vi "Lift Control (SubVI).vi"(10 "Buttons":bool[](array[boolean]), 11 "Lift PID gains":T1={"proportional gain (Kc)"=1.0, "integral time (Ti, min)"=0.01, "derivative time (Td, min)"=0.0} {"derivative time (Td, min)" format="%.3f"; "integral time (Ti, min)" format="%.3f"; "proportional gain (Kc)" format="%.3f"}) -> ()   [LabVIEW 2014]
uses:
  <vilib>/Rock Robotics/WPI/Solenoid/WPI_SolenoidValue.ctl
  <vilib>/Rock Robotics/WPI/Solenoid/WPI_SolenoidSetEnum.vi
  <vilib>/addons/control/pid/pid.llb/PID (DBL).vi
  <vilib>/addons/control/pid/NI_PID_pid.lvlib
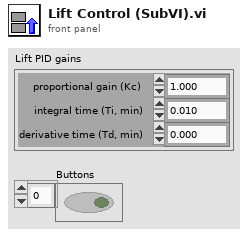
[diagram p1: front panel]
types:
  T1 = cluster{"proportional gain (Kc)":dbl, "integral time (Ti, min)":dbl, "derivative time (Td, min)":dbl}
  T2 = typedef "WPI_SolenoidValue.ctl" = enum16{"Off", "On", "Forward", "Reverse"}
  T3 = typedef "WPI_EncoderDevRef.ctl" = cluster{"DevStatus":errorcluster, "EncoderIndex":T4, "CounterIndex":T5, "DistancePerCount":dbl, "Decoding Type":T6}
  T4 = typedef "FPGA_EncoderIdx.ctl" = enum8{"Enc 0", "Enc 1", "Enc 2", "Enc 3", "Enc 4", "Enc 5", "Enc 6", "Enc 7", "Invalid"}
  T5 = typedef "FPGA_CounterCtrSystemIndex.ctl" = enum8{"Ctr 0", "Ctr 1", "Ctr 2", "Ctr 3", "Ctr 4", "Ctr 5", "Ctr 6", "Ctr 7", "Invalid"}
  T6 = typedef "WPI_EncoderType.ctl" = enum16{"1x", "2x", "4x"}
  T7 = typedef "WPI_SolenoidDevRef.ctl" = cluster{"DevStatus":errorcluster, "Pneumatics Control Module":u8, "Forward Solenoid Channel":T8, "Reverse Solenoid Channel":T8}
  T8 = typedef "WPI_SolenoidChannel.ctl" = enum8{"Solenoid 0", "Solenoid 1", "Solenoid 2", "Solenoid 3", "Solenoid 4", "Solenoid 5", "Solenoid 6", "Solenoid 7", "Invalid"}
  T9 = typedef "WPI_SwitchDevRef.ctl" = cluster{"DevStatus":errorcluster, "DIO Channel":T10, "Controller":T11, "CntIndex":T5, "Normally Closed":bool}
  T10 = typedef "FPGA_DIOChannel.ctl" = enum8{"DIO 0", "DIO 1", "DIO 2", "DIO 3", "DIO 4", "DIO 5", "DIO 6", "DIO 7", "DIO 8", "DIO 9", "DIO MXP 0", "DIO MXP 1", "DIO MXP 2", "DIO MXP 3", "DIO MXP 4", "DIO MXP 5", "DIO MXP 6", "DIO MXP 7", "DIO MXP 8", "DIO MXP 9", "DIO MXP 10", "DIO MXP 11", "DIO MXP 12", "DIO MXP 13", "DIO MXP 14", "DIO MXP 15", "Invalid"}
  T11 = typedef "FPGA_TypedefDigitalModule.ctl" = enum16{"Controller 1"}
  T12 = typedef "WPI_MotorControlDeviceRef.ctl" = cluster{"DeviceStatus":errorcluster, "Type":T13, "PWM":cluster{"Controller":T11, "PWM Channel":T14, "DeadBand":T15}, "CAN":cluster{"Device Number":u8, "Control Mode":T16, "Semaphore":T17, "Max Vout":dbl, "TalonSRX Control Mode":T18}, "Invert":bool, "TransformRef":T19, "InvTransformRef":T19}
  T13 = typedef "WPI_MotorControlType.ctl" = enum16{"PWM", "CAN", "CANTalonSRX"}
  T14 = typedef "FPGA_DIOPWMChannel.ctl" = enum8{"PWM 0", "PWM 1", "PWM 2", "PWM 3", "PWM 4", "PWM 5", "PWM 6", "PWM 7", "PWM 8", "PWM 9", "PWM MXP 0", "PWM MXP 1", "PWM MXP 2", "PWM MXP 3", "PWM MXP 4", "PWM MXP 5", "PWM MXP 6", "PWM MXP 7", "PWM MXP 8", "PWM MXP 9", "Invalid"}
  T15 = typedef "WPI_PWMDeadband.ctl" = cluster{"Name":string, "maxPositivePwm":i32, "minPositivePwm":i32, "centerPwm":i32, "maxNegativePwm":i32, "minNegativePwm":i32, "angularRange":u16}
  T16 = typedef "WPI_CANJaguar_ControlMode.ctl" = enum8{"Percent VBus", "Current", "Speed", "Position", "Voltage"}
  T17 = typedef "Semaphore RefNum" = refnum<k1>
  T18 = typedef "WPI_CANTalonSRX_APIControlMode.ctl" = enum8{"Percent VBus", "Speed", "Position", "Slave", "Unchanged / Invalid"}
  T19 = typedef "WPI_PWMTransform_ConPane.ctl" = refnum<vi>
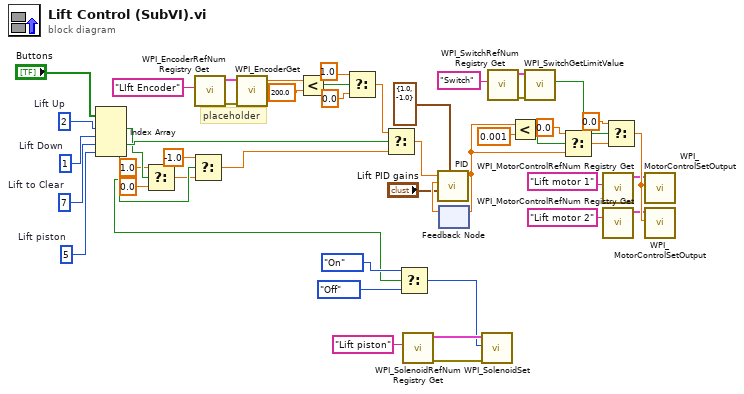
[diagram p0: block diagram]
diagram:
  w1 = 5  # Lift piston
  w47 = 7  # Lift to Clear
  w45 = 1  # Lift Down
  w43 = 2  # Lift Up
  # "placeholder"
  n1 = Index Array(array="Buttons", index #1=w43, index #2=w45, index #3=w47, index #4=w1) -> (element #1=w44:bool, element #2=w46:bool, element #3=w48:bool, element #4=w3:bool)
  n2 = Select(t=1.0, s=w44, f=0.0) -> (s? t:f=w17:dbl)
  n3 = Select(t=-1.0 ("f"), s=w46, f=w17) -> (s? t:f=w27:dbl)
  n4 = call <vilib>:"WPI_EncoderRefNum Registry Get.vi"("refnum name"="LIft Encoder") -> ("error out"=w26:errorcluster, "EncoderDevRef"=w25:T3)  [unwired: 9 in]
  n5 = call <vilib>:"WPI_EncoderGet.vi"("error in (no error)"=w26, "EncoderDevRef"=w25) -> ("Distance"=w29:dbl)  [unwired: 4 in, 5 out]
  n6 = Less?(x=w29, y=200.0) -> (x < y?=w31:bool)
  n7 = Select(t=1.0, s=w31, f=0.0) -> (s? t:f=w33:dbl)
  n8 = Select(t=w33, s=w48, f=w27) -> (s? t:f=w28:dbl)
  n9 = Select(t=WPI_SolenoidValue."On" ("Value"), s=w3, f=WPI_SolenoidValue."Off" ("Value")) -> (s? t:f=w2:T2)
  n10 = call <vilib>:"WPI_SolenoidRefNum Registry Get.vi"("refnum name"="Lift piston") -> ("error out"=w8:errorcluster, "SolenoidDevRef"=w7:T7)  [unwired: 9 in]
  n11 = feedback #1() -> (w24:dbl)  [unwired: 1 in]
  n12 = call-poly <vilib>:"PID.vi"("output range"=cluster{"output high":dbl, "output low":dbl} {"output high"=1.0, "output low"=-1.0}, "PID gains"="Lift PID gains", "process variable"=w24, "setpoint"=w28) -> ("output"=w23:dbl)  [unwired: 6 in, 1 out]
  n13 = feedback-in #1(w23) -> ()
  n14 = call-poly <vilib>:"WPI_SolenoidSet.vi"("error in (no error)"=w8, "Value"=w2, "SolenoidDevRef"=w7) -> ()  [unwired: 7 in, 2 out]
  n15 = call <vilib>:"WPI_SwitchRefNum Registry Get.vi"("refnum name"="Switch") -> ("error out"=w35:errorcluster, "SwitchDevRef"=w36:T9)  [unwired: 9 in]
  n16 = Less?(x=w23, y=0.001) -> (x < y?=w21:bool)
  n17 = call <vilib>:"WPI_SwitchGetLimitValue.vi"("error in (no error)"=w35, "SwitchDevRef"=w36) -> ("Switch Pressed"=w38:bool)  [unwired: 7 in, 2 out]
  n18 = Select(t=0.0, s=w21, f=w23) -> (s? t:f=w39:dbl)
  n19 = call <vilib>:"WPI_MotorControlRefNum Registry Get.vi"("refnum name"="Lift motor 1") -> ("MotorControlDevRef"=w18:T12)  [unwired: 9 in, 1 out]
  n20 = call <vilib>:"WPI_MotorControlRefNum Registry Get.vi"("refnum name"="Lift motor 2") -> ("MotorControlDevRef"=w15:T12)  [unwired: 9 in, 1 out]
  n21 = Select(t=0.0, s=w38, f=w39) -> (s? t:f=w40:dbl)
  n22 = call <vilib>:"WPI_MotorControlSetOutput.vi"("Output"=w40, "MotorControlDevRef"=w18) -> ()  [unwired: 7 in, 3 out]
  n23 = call <vilib>:"WPI_MotorControlSetOutput.vi"("Output"=w40, "MotorControlDevRef"=w15) -> ()  [unwired: 7 in, 3 out]
